vi "pcap-init.vi"() -> (2 "error_string":string, 3 "return type":i32)   [LabVIEW 2017]
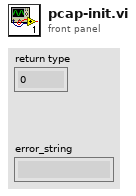
[diagram p1: front panel]
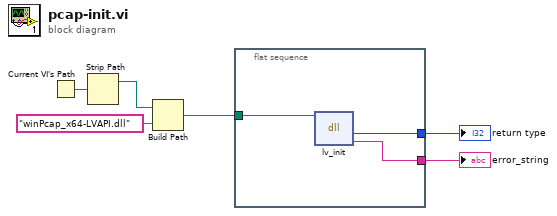
[diagram p0: block diagram]
diagram:
  n1 = Current VI's Path() -> (path=w6:path)
  n2 = Strip Path(path=w6) -> (stripped path=w5:path)  [unwired: 1 out]
  n3 = Build Path(base path=w5, name or relative path="winPcap_x64-LVAPI.dll") -> (appended path=w3:path)
  n4 = flat-sequence {
    tunnel: w3 -> [w9]
    tunnel: [w8] -> w2
    tunnel: [w7] -> w1
    frame #0 {
      n5 = dll-call lib="C:/Users/ucbtspu.AD/OneDrive - University College London/Local SCC/SilverLab-Microscope x64/Ethernet/winPcap_x64-LVAPI.dll" fn="lv_init"(path in=w9) -> ("return type"=w7:i32, "error_string"=w8:string)  [unwired: 3 in, 2 out]
    }
  }
  "error_string" <- w2
  "return type" <- w1
